vi "Status.vi"(10 "ModuleList":string[](array[string])=["Sync", "FGen", "Digitizer", "Sensor", "Analysis", "Scope", "AcPwr"]) -> ()   [LabVIEW 2018, in "Visualization.lvlib" / "VisualizeStatus.lvclass"]
uses:
  VisualizeStatus.lvclass
  VisualizeBase/VisualizeBase_class/Requests/VisUserEventType.ctl
  <vilib>/event_ctls.llb/usereventprio.ctl
  <extravilib>/ChannelInstances/Tag-bool/Read With Abort.vi
  <extravilib>/ChannelInstances/Tag-bool/Write With Abort.vi
  <vilib>/Utility/error.llb/Error Cluster From Error Code.vi
  <extravilib>/ChannelInstances/Tag-bool/Instantiate.vi
  <extravilib>/ChannelInstances/Tag-bool/EndpointRead.vi
  <extravilib>/ChannelInstances/Tag-bool/Endpoint.vi
  <vilib>/ErrorRing/Error Ring.xnode
  VisualizeBase/VisualizeBase_class/VisualizeBase.lvclass
  <userlib>/NIST/NISTErrorLib/NISTErrorLib.lvlib
  Sync/SyncModule/SyncModule.lvlib
  Digitizer/DigitizerModule/DigitizerModule.lvlib
  BusClass/Bus.lvclass
  Sensor/SensorModule/SensorModule.lvlib
  Analysis/AnalysisModule/AnalysisModule.lvlib
  Scope/ScopeModule/ScopeModule.lvlib
  AcPwr/AcPwrShared/AcPwrShared.lvlib
  <extravilib>/ChannelInstances/Tag-bool.lvlib
  TestClass/Test.lvclass
  FGen/FgenShared/FgenShared.lvlib
panel:
  out "Status Message":string
  out "ErrorArray":errorcluster[](array[cluster])
  in  "btnReset":bool
  in  "btnClear":bool
  in  "QueName":string="StatusVisQue"
  in  "btnStop&Exit":bool
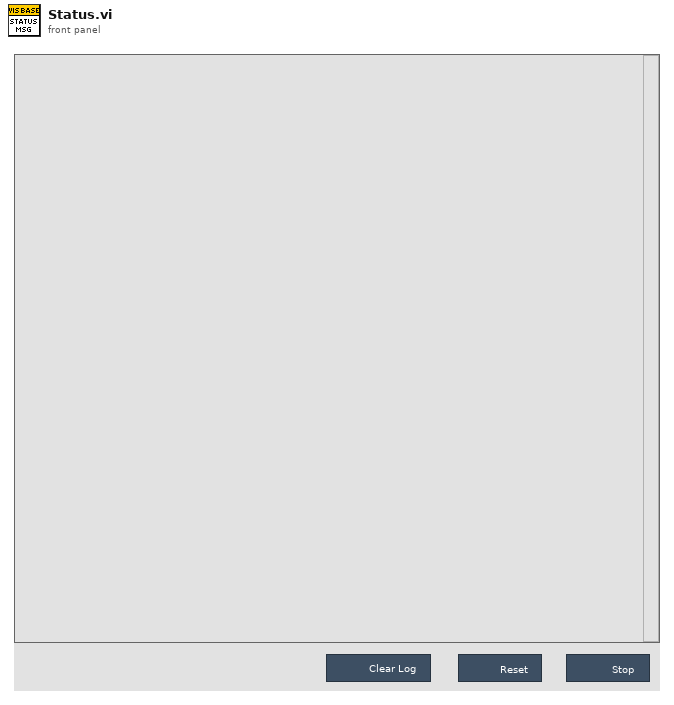
[diagram p1: front panel]
types:
  T1 = typedef "SyncModule.lvlib/SyncBroadcastEvents.ctl" = cluster{"DidInit":refnum<user-event>, "StatusUpdate":refnum<user-event>, "ErrorReport":refnum<user-event>, "DidStop":refnum<user-event>, "PathToINI":refnum<user-event>, "TriggerTime":refnum<user-event>, "LockStatus":refnum<user-event>, "Info":refnum<user-event>, "ClockProperties":refnum<user-event>, "SyncData":refnum<user-event>}
  T2 = typedef "AcPwrShared.lvlib/AcPwrBroadcastEvents.ctl" = cluster{"DidInit":refnum<user-event>, "StatusUpdate":refnum<user-event>, "ErrorReport":refnum<user-event>, "DidStop":refnum<user-event>, "PathToINI":refnum<user-event>, "Measurements":refnum<user-event>, "LoadConfigFile":refnum<user-event>, "GetSettings":refnum<user-event>, "SetSettings":refnum<user-event>, "GetType&ID":refnum<user-event>, "GotSettings":refnum<user-event>}
  T3 = typedef "FgenShared.lvlib/clBroadcastEvents.ctl" = cluster{"DidInit":refnum<user-event>, "StatusUpdate":refnum<user-event>, "ErrorReport":refnum<user-event>, "DidStop":refnum<user-event>, "PathToINI":refnum<user-event>, "Channels":refnum<user-event>, "Function":refnum<user-event>, "Waveforms":refnum<user-event>, "Triggers":refnum<user-event>, "FunctionParams":refnum<user-event>, "FunctionArbs":refnum<user-event>, "FunctionSampleRate":refnum<user-event>}
  T4 = typedef "ScopeShared.lvlib/clBroadcastEvents.ctl" = cluster{"DidInit":refnum<user-event>, "StatusUpdate":refnum<user-event>, "ErrorReport":refnum<user-event>, "DidStop":refnum<user-event>, "PathToINI":refnum<user-event>, "Handle":refnum<user-event>, "Model":refnum<user-event>, "Channels":refnum<user-event>, "Acquisition":refnum<user-event>, "Trigger":refnum<user-event>, "ExtAcquisition":refnum<user-event>, "Waveform":refnum<user-event>}
  T5 = typedef "DigitizerShared.lvlib/clBroadcastEvents.ctl" = cluster{"DidInit":refnum<user-event>, "StatusUpdate":refnum<user-event>, "ErrorReport":refnum<user-event>, "DidStop":refnum<user-event>, "PathToINI":refnum<user-event>, "Channels":refnum<user-event>, "Acq":refnum<user-event>, "Trigger":refnum<user-event>, "Waveforms":refnum<user-event>}
  T6 = typedef "SensorShared.lvlib/clBroadcastEvents.ctl" = cluster{"DidInit":refnum<user-event>, "StatusUpdate":refnum<user-event>, "ErrorReport":refnum<user-event>, "DidStop":refnum<user-event>, "PathToINI":refnum<user-event>, "SensorReport":refnum<user-event>, "SensorConfig":refnum<user-event>}
  T7 = typedef "AnalysisModule.lvlib/clBroadcastEvents.ctl" = cluster{"DidInit":refnum<user-event>, "StatusUpdate":refnum<user-event>, "ErrorReport":refnum<user-event>, "DidStop":refnum<user-event>, "PathToINI":refnum<user-event>, "Config":refnum<user-event>, "ResultReport":refnum<user-event>, "FunctionClass":refnum<user-event>, "State":refnum<user-event>, "FunctionParams":refnum<user-event>, "Duration":refnum<user-event>}
  T8 = cluster{"DigitizerEvents":T5, "FGenEvents":T3, "SyncBroadcastEvents":T1, "AnalysisBroadcastEvents":T7, "SensorBdcstEvents":T6, "ScopeEvents":T4, "clAcPwrEvents":T2}
  T9 = cluster{"StatusUpdate":refnum<user-event>, "ErrorReport":refnum<user-event>, "StatusUpdate":refnum<user-event>, "ErrorReport":refnum<user-event>, "StatusUpdate":refnum<user-event>, "ErrorReport":refnum<user-event>, "StatusUpdate":refnum<user-event>, "ErrorReport":refnum<user-event>, "StatusUpdate":refnum<user-event>, "ErrorReport":refnum<user-event>, "StatusUpdate":refnum<user-event>, "ErrorReport":refnum<user-event>, "FunctionClass":refnum<user-event>, "StatusUpdate":refnum<user-event>, "ErrorReport":refnum<user-event>}
  T10 = typedef "clUserEvents.ctl" = cluster{"StopEvent":refnum<user-event>, "RefreshUserEvents":refnum<user-event>, "StatusUpdate":refnum<user-event>, "RunAllScripts":refnum<user-event>}
  T11 = typedef "Visualization.lvlib/VisualizeBase.lvclass/VisRequestEvents.ctl" = cluster{"StopRequest":refnum<user-event>, "ResetRequest":refnum<user-event>, "FP Pop In or Out":refnum<user-event>}
  T12 = typedef "Visualization.lvlib/VisualizeBase.lvclass/VisUserEventType.ctl" = cluster{"BusIndex":i8, "Data":variant}
  T13 = typedef "usereventprio.ctl" = enum32{"high priority", "normal priority"}
  T14 = typedef "Tag-bool.lvlib/))Channel.ctl" = refnum<queue>
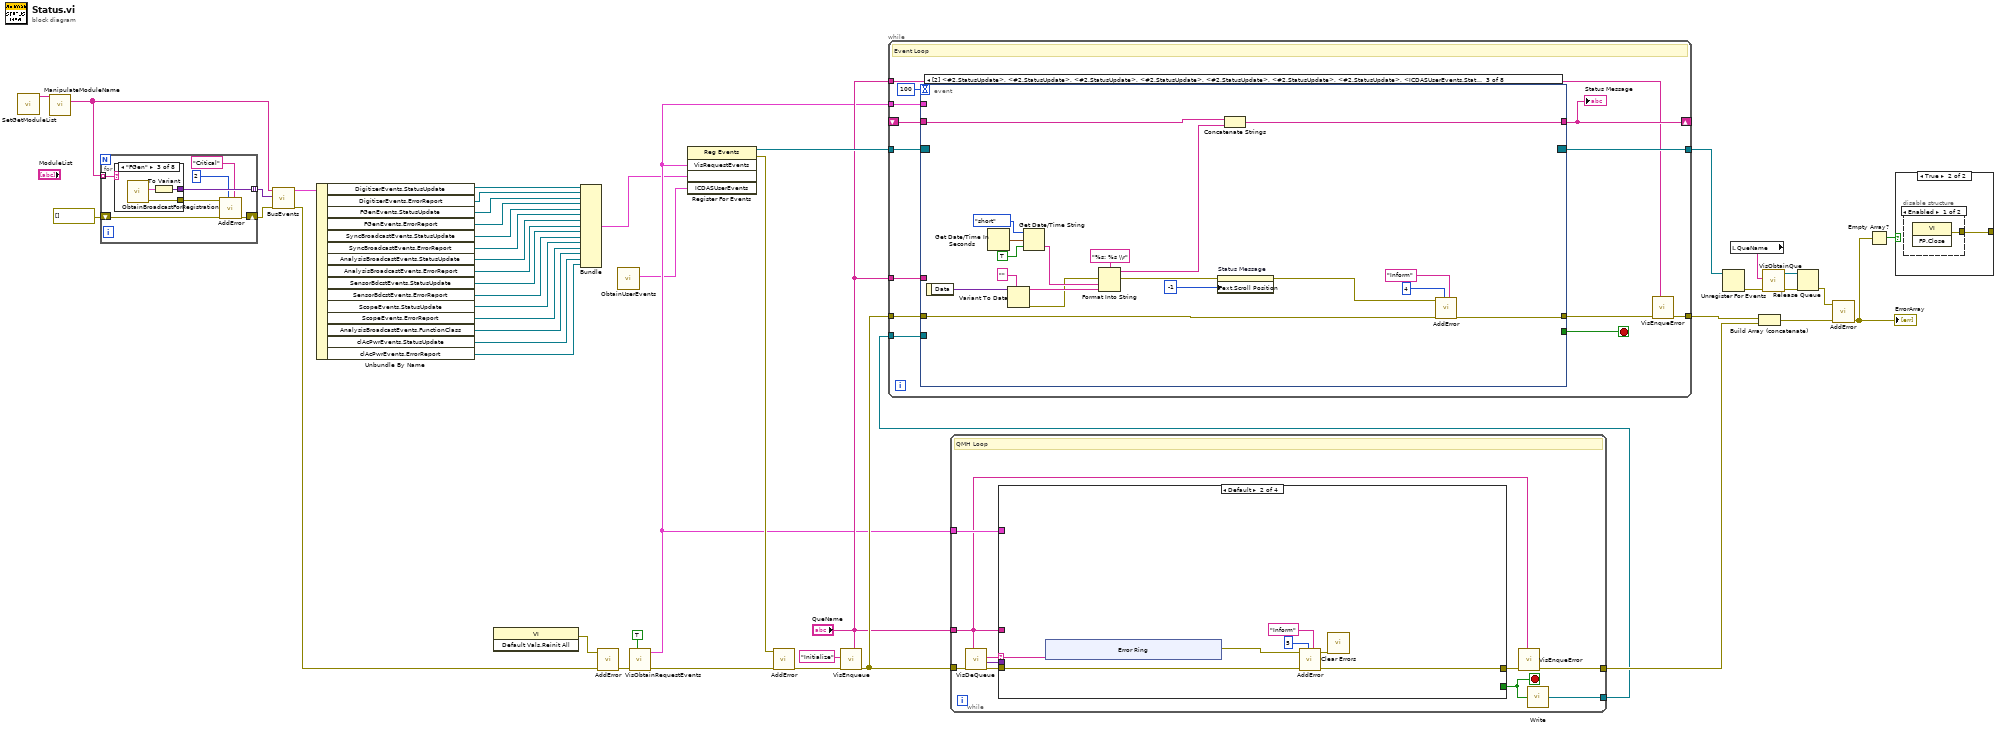
[diagram p0: block diagram]
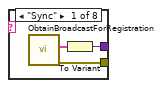
[diagram p2: hidden frame]
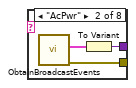
[diagram p3: hidden frame]
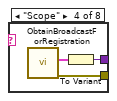
[diagram p4: hidden frame]
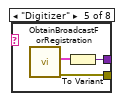
[diagram p5: hidden frame]
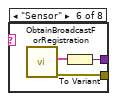
[diagram p6: hidden frame]
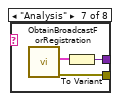
[diagram p7: hidden frame]
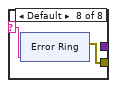
[diagram p8: hidden frame]
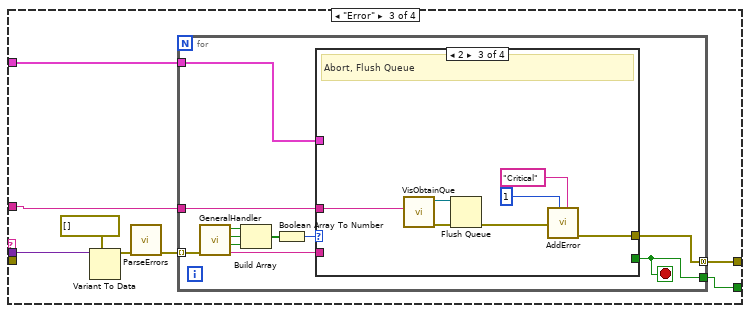
[diagram p10: hidden frame]
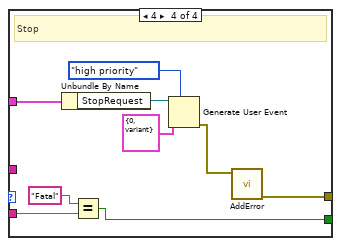
[diagram p13: hidden frame]
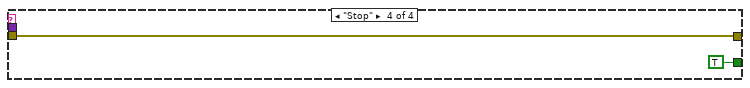
[diagram p14: hidden frame]
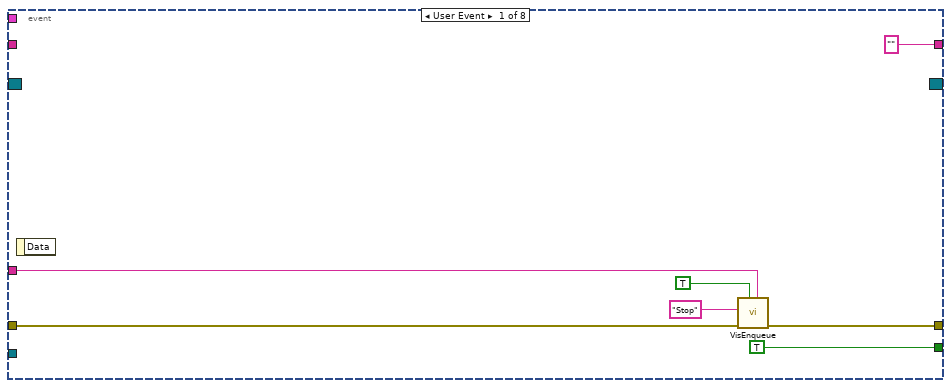
[diagram p15: hidden frame]
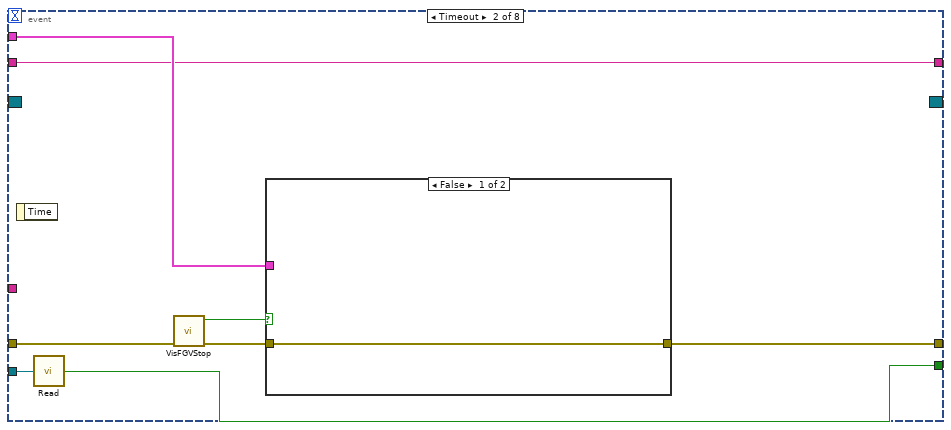
[diagram p16: hidden frame]
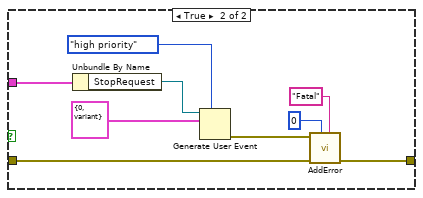
[diagram p17: hidden frame]
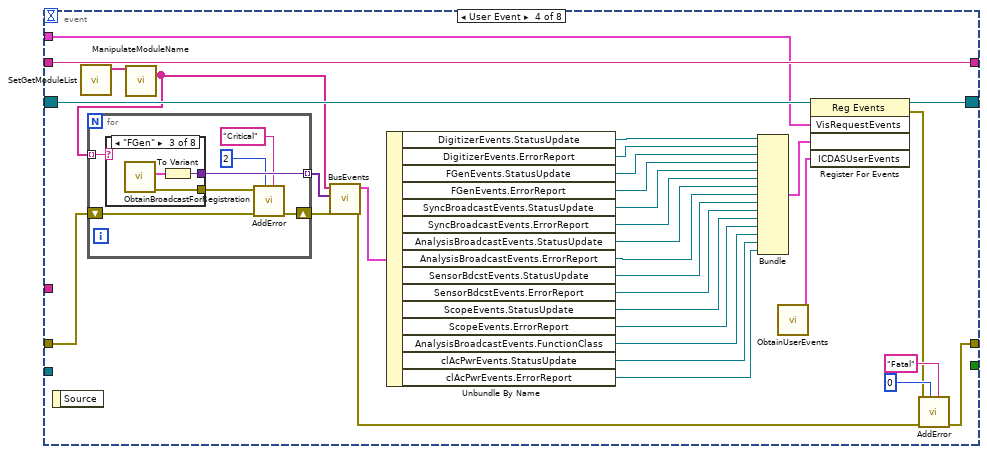
[diagram p18: hidden frame]
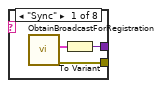
[diagram p19: hidden frame]
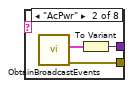
[diagram p20: hidden frame]
diagram:
  n1 = call "SetGetModuleList.vi"() -> ("ModuleList"=w24:string[])  [unwired: 11 in]
  n2 = call "ManipulateModuleName.vi"("ModuleListArrayIn"=w24) -> ("BeforeMatch:ModuleListArray"=w19:string[])  [unwired: 9 in, 5 out]
  n3 = for {
    shift-right: [w52] -> w21
    shift-left: errorcluster[] [] ("ErrorArray") -> [w51]
    tunnel: [w50] -> w20 mode=indexing
    tunnel: w19 -> [w47] mode=indexing
    n4 = case shown="\"FGen\"" w47 {
      selector: w47 -> [_ _ _ _ _ _ _ w75]
      tunnel: [w55 w59 w61 w63 w67 w70 w73 _] -> w50
      tunnel: [w54 w58 w62 w65 w68 w71 w74 w76] -> w53
      frame "Sync" {
        n5 = call "ObtainBroadcastForRegistration.vi"() -> ("error out"=w54:errorcluster, "SyncBroadcastEvents"=w56:T1)  [unwired: 10 in]
        n6 = To Variant(anything=w56) -> (Variant=w55:variant)
      }
      frame "AcPwr" {
        n7 = call "ObtainBroadcastEvents.vi"() -> ("error out"=w58:errorcluster, "clAcPwrEvents"=w57:T2)  [unwired: 10 in]
        n8 = To Variant(anything=w57) -> (Variant=w59:variant)
      }
      frame "FGen" {
        n9 = call "ObtainBroadcastForRegistration.vi"() -> ("error out"=w62:errorcluster, "FgenBroadcastEvents"=w60:T3)  [unwired: 10 in]
        n10 = To Variant(anything=w60) -> (Variant=w61:variant)
      }
      frame "Scope" {
        n11 = call "ObtainBroadcastForRegistration.vi"() -> ("error out"=w65:errorcluster, "ScopeBroadcastEvents"=w64:T4)  [unwired: 10 in]
        n12 = To Variant(anything=w64) -> (Variant=w63:variant)
      }
      frame "Digitizer" {
        n13 = call "ObtainBroadcastForRegistration.vi"() -> ("error out"=w68:errorcluster, "clDigitizerBdcstEvents"=w66:T5)  [unwired: 10 in]
        n14 = To Variant(anything=w66) -> (Variant=w67:variant)
      }
      frame "Sensor" {
        n15 = call "ObtainBroadcastForRegistration.vi"() -> ("error out"=w71:errorcluster, "SensorBdcstEvents"=w69:T6)  [unwired: 10 in]
        n16 = To Variant(anything=w69) -> (Variant=w70:variant)
      }
      frame "Analysis" {
        n17 = call "ObtainBroadcastForRegistration.vi"() -> ("error out"=w74:errorcluster, "AnalysisBroadcastEvents"=w72:T7)  [unwired: 10 in]
        n18 = To Variant(anything=w72) -> (Variant=w73:variant)
      }
      frame Default {
        n19 = xnode "Error Ring"("parameter 0"=w75) -> ("error out"=w76:errorcluster)
      }
    }
    n20 = call <userlib>:"AddError.vi"("Severity"="Critical", "Priority"=u8 2, "ErrorArray In"=w51, "error in (no error)"=w53) -> ("ErrorArray Out"=w52:errorcluster[])  [unwired: 6 in, 1 out]
  }
  n21 = call "BusEvents.vi"("Error in"=w21, "EventArray"=w20, "ModuleList"=w19) -> ("output cluster"=w18:T8)  [unwired: 7 in, 1 out]
  n22 = Unbundle By Name(w18) -> ("DigitizerEvents.StatusUpdate"=w17:refnum<user-event>, "DigitizerEvents.ErrorReport"=w16:refnum<user-event>, "FGenEvents.StatusUpdate"=w15:refnum<user-event>, "FGenEvents.ErrorReport"=w14:refnum<user-event>, "SyncBroadcastEvents.StatusUpdate"=w13:refnum<user-event>, "SyncBroadcastEvents.ErrorReport"=w12:refnum<user-event>, "AnalysisBroadcastEvents.StatusUpdate"=w11:refnum<user-event>, "AnalysisBroadcastEvents.ErrorReport"=w10:refnum<user-event>, "SensorBdcstEvents.StatusUpdate"=w9:refnum<user-event>, "SensorBdcstEvents.ErrorReport"=w8:refnum<user-event>, "ScopeEvents.StatusUpdate"=w7:refnum<user-event>, "ScopeEvents.ErrorReport"=w6:refnum<user-event>, "AnalysisBroadcastEvents.FunctionClass"=w5:refnum<user-event>, "clAcPwrEvents.StatusUpdate"=w4:refnum<user-event>, "clAcPwrEvents.ErrorReport"=w3:refnum<user-event>)
  n23 = invoke class="VI" method="Default Vals.Reinit All"() -> (error out=w45:errorcluster)  [unwired: 3 in, 2 out]
  n24 = Bundle("StatusUpdate"=w17, "ErrorReport"=w16, "StatusUpdate"=w15, "ErrorReport"=w14, "StatusUpdate"=w13, "ErrorReport"=w12, "StatusUpdate"=w11, "ErrorReport"=w10, "StatusUpdate"=w9, "ErrorReport"=w8, "StatusUpdate"=w7, "ErrorReport"=w6, "FunctionClass"=w5, "StatusUpdate"=w4, "ErrorReport"=w3) -> (w2:T9)  [unwired: 1 in]
  n25 = call <userlib>:"AddError.vi"("ErrorArray In"=w21, "error in (no error)"=w45) -> ("ErrorArray Out"=w44:errorcluster[])  [unwired: 8 in, 1 out]
  n26 = call "ObtainUserEvents.vi"() -> ("ICDASUserEvents"=w22:T10)  [unwired: 10 in, 1 out]
  n27 = call "VisObtainRequestEvents.vi"("Set (T)/Get (F)"=TRUE, "Error"=w44) -> ("Error"=w43:errorcluster[], "VisRequestEvents"=w25:T11)  [unwired: 8 in]
  n28 = register-events(w25, w2, w22) -> (reference out=w31:refnum<event-registration>, error out=w30:errorcluster)  [unwired: 2 in]
  n29 = call <userlib>:"AddError.vi"("ErrorArray In"=w43, "error in (no error)"=w30) -> ("ErrorArray Out"=w32:errorcluster[])  [unwired: 8 in, 1 out]
  n30 = call "VisEnqueue.vi"("QueName"="QueName", "Error"=w32, "Message"="Initialize") -> ("Error"=w28:errorcluster[])  [unwired: 8 in]
  n31 = while {
    tunnel: w28 -> [w93]
    tunnel: [w87] -> w40
    tunnel: w25 -> [w86]
    tunnel: "QueName" -> [w85]
    tunnel: [w84] -> w26
    stop <- w88 stop-if-true
    # "QMH Loop"
    n32 = call "VisDeQueue.vi"("QueName"=w85, "Error"=w93) -> ("Error"=w90:errorcluster[], "Data"=w91:variant, "Message"=w92:string)  [unwired: 7 in]
    n33 = case shown="Default" w92 {
      selector: w92 -> [_ w101 _ _]
      tunnel: w91 -> [_ _ w116 _]
      tunnel: w90 -> [w94 w99 _ w144]
      tunnel: [w94 w98 w112 w144] -> w89
      tunnel: [_ _ w111 TRUE] -> w88
      tunnel: w86 -> [_ _ w110 _]
      tunnel: w85 -> [_ _ w109 _]
      frame "Initialize" {
      }
      frame Default {
        n34 = xnode "Error Ring"("parameter 0"=w101) -> ("error out"=w100:errorcluster)
        n35 = call <userlib>:"AddError.vi"("Severity"="Inform" ("String"), "Priority"=u8 5, "ErrorArray In"=w99, "error in (no error)"=w100) -> ("ErrorArray Out"=w98:errorcluster[], "error out"=w97:errorcluster)  [unwired: 6 in]
        n36 = call <vilib>:"Clear Errors.vi"("error in (no error)"=w97) -> ()  [unwired: 5 in, 2 out]
      }
      frame "Error" {
        n37 = Variant To Data(type=errorcluster[] [], Variant=w116) -> (data=w114:errorcluster[])  [unwired: 1 in, 1 out]
        n38 = call <userlib>:"ParseErrors.vi"("ErrorArray"=w114) -> ("ErrorArray"=w113:errorcluster[])  [unwired: 8 in, 2 out]
        n39 = for {
          tunnel: w113 -> [w127] mode=indexing
          tunnel: [w121] -> w112 mode=concatenating
          tunnel: [w119] -> w111
          tunnel: w110 -> [w118]
          tunnel: w109 -> [w117]
          stop <- w119 stop-if-true
          n40 = call <userlib>:"GeneralHandler.vi"("error in (no error)"=w127) -> ("Severity"=w120:string, "Stop"=w124:bool, "Abort"=w125:bool, "Continue"=w126:bool)  [unwired: 6 in, 1 out]
          n41 = Build Array(w126, w125, w124) -> (w123:bool[])
          n42 = Boolean Array To Number(Boolean array=w123) -> (number=w122:u32)
          n43 = case shown="2" w122 {
            tunnel: [_ _ w132 w142] -> w121
            tunnel: w120 -> [_ _ _ w138]
            tunnel: [_ _ _ w136] -> w119
            tunnel: w118 -> [_ _ _ w135]
            tunnel: w117 -> [_ _ w128 _]
            frame 0, Default {
              # "No Dialog"
            }
            frame 1 {
              # "Continue"
            }
            frame 2 {
              # "Abort, Flush Queue"
              n44 = call "VisObtainQue.vi"("QueName"=w128) -> ("error out"=w134:errorcluster, "queue out"=w133:refnum<queue>)  [unwired: 9 in]
              n45 = Flush Queue(queue=w133, error in (no error)=w134) -> (error out=w131:errorcluster)  [unwired: 2 out]
              n46 = call <userlib>:"AddError.vi"("Severity"="Critical" ("String"), "Priority"=u8 1, "error in (no error)"=w131) -> ("ErrorArray Out"=w132:errorcluster[])  [unwired: 7 in, 1 out]
            }
            frame 4 {
              # "Stop"
              n47 = Unbundle By Name(w135) -> ("StopRequest"=w143:refnum<user-event>)
              n48 = Equal?(x="Fatal", y=w138) -> (x = y?=w136:bool)
              n49 = Generate User Event(priority (normal)=usereventprio."high priority", user event=w143, event data cluster=T12 {"BusIndex"=0, "Data"=variant} ("event data")) -> (error out=w141:errorcluster)  [unwired: 1 in, 1 out]
              n50 = call <userlib>:"AddError.vi"("error in (no error)"=w141) -> ("ErrorArray Out"=w142:errorcluster[])  [unwired: 9 in, 1 out]
            }
          }
        }
      }
      frame "Stop" {
      }
    }
    n51 = call "VisEnqueError.vi"("QueName"=w85, "Error"=w89) -> ("Error"=w87:errorcluster[])  [unwired: 9 in]
    n52 = call <extravilib>:"Write.vi"("element"=w88) -> ("channel"=w84:T14)  [unwired: 1 out]
  }
  n53 = while {
    tunnel: w31 -> [w158]
    tunnel: [w155] -> w41
    tunnel: [w154] -> w42
    tunnel: w25 -> [w153]
    shift-right: [w150] -> _
    shift-left: _ -> [w152]
    tunnel: w28 -> [w151]
    tunnel: "QueName" -> [w149]
    tunnel: "QueName" -> [w148]
    tunnel: w26 -> [w146]
    stop <- w157 stop-if-true
    # "Event Loop"
    n54 = event shown="[2] <#2.StatusUpdate>, <#2.StatusUpdate>, <#2.StatusUpdate>, <#2.StatusUpdate>, <#2.StatusUpdate>, <#2.StatusUpdate>, <#2.StatusUpdate>, <ICDASUserEvents.StatusUpdate>: User Event" {
      selector: w158 -> [_ _ _ w229 _ _ _ _]
      dyn-events: [_ _ _ w231 _ _ _ _] -> w154
      timeout: 100 -> [_ _ _ _ _ _ _ _]
      tunnel: [TRUE w166 _ _ _ _ _ _] -> w157
      tunnel: [w164 w172 w194 w234 w281 _ w300 w306] -> w156
      tunnel: w153 -> [_ w169 _ w222 _ _ w295 w305]
      tunnel: ["" w168 w190 w227 w276 "" w293 w303] -> w150
      tunnel: w152 -> [_ w168 w189 w227 w275 _ w293 w303]
      tunnel: w151 -> [w160 w171 w188 w228 w272 _ w294 w304]
      tunnel: w148 -> [w161 _ _ _ _ _ _ _]
      tunnel: w146 -> [_ w167 _ _ _ _ _ _]
      event User Event {
        n55 = event-data() -> ()  [unwired: 1 in, 1 out]
        n56 = call "VisEnqueue.vi"("QueName"=w161, "Priority? (F)"=TRUE, "Error"=w160, "Message"="Stop") -> ("Error"=w164:errorcluster[])  [unwired: 7 in]
      }
      event Timeout {
        n57 = event-data() -> ()  [unwired: 1 in, 1 out]
        n58 = call <extravilib>:"Read.vi"("channel"=w167) -> ("element"=w166:bool)  [unwired: 1 in, 1 out]
        n59 = call "VisFGVStop.vi"("Error In"=w171) -> ("Error Out"=w170:errorcluster[], "Value"=w173:bool)  [unwired: 9 in]
        n60 = case shown="False" w173 {
          tunnel: [w174 w177] -> w172
          tunnel: w170 -> [w174 w176]
          tunnel: w169 -> [_ w175]
          frame False {
          }
          frame True {
            n61 = Unbundle By Name(w175) -> ("StopRequest"=w183:refnum<user-event>)
            n62 = Generate User Event(priority (normal)=usereventprio."high priority", user event=w183, event data cluster=T12 {"BusIndex"=0, "Data"=variant} ("event data")) -> (error out=w178:errorcluster)  [unwired: 1 in, 1 out]
            n63 = call <userlib>:"AddError.vi"("Severity"="Fatal" ("String"), "Priority"=u8 0, "ErrorArray In"=w176, "error in (no error)"=w178) -> ("ErrorArray Out"=w177:errorcluster[])  [unwired: 6 in, 1 out]
          }
        }
      }
      event User Event {
        n64 = event-data() -> ("Data"=w184:variant)  [unwired: 1 in]
        n65 = Get Date/Time In Seconds() -> (seconds since 1Jan1904=w202:timestamp)
        n66 = Variant To Data(type="", Variant=w184) -> (data=w196:string, error out=w195:errorcluster)  [unwired: 1 in]
        n67 = Get Date/Time String(date format (0)=enum16{"short", "long", "abbreviated"}."short", seconds (now)=w202, want seconds? (F)=TRUE) -> (time string=w197:string)  [unwired: 1 out]
        n68 = Format Into String(format string="%s: %s \\r", error in=w195, w197, w196) -> (resulting string=w191:string, error out=w187:errorcluster)  [unwired: 1 in]
        n69 = property on="Status Message" class="Str"(error in=w187, "Text.Scroll Position"=-1) -> (error out=w186:errorcluster)  [unwired: 1 in, 1 out]
        n70 = Concatenate Strings(w189, w191) -> (w190:string)
        n71 = call <userlib>:"AddError.vi"("Severity"="Inform", "Priority"=u8 4, "ErrorArray In"=w188, "error in (no error)"=w186) -> ("ErrorArray Out"=w194:errorcluster[])  [unwired: 6 in, 1 out]
      }
      event User Event {
        n72 = event-data() -> ()  [unwired: 1 in, 1 out]
        n73 = call "SetGetModuleList.vi"() -> ("ModuleList"=w226:string[])  [unwired: 11 in]
        n74 = call "ManipulateModuleName.vi"("ModuleListArrayIn"=w226) -> ("BeforeMatch:ModuleListArray"=w203:string[])  [unwired: 9 in, 5 out]
        n75 = for {
          shift-right: [w240] -> w223
          shift-left: w228 -> [w239]
          tunnel: [w238] -> w225 mode=indexing
          tunnel: w203 -> [w235] mode=indexing
          n76 = case shown="\"FGen\"" w235 {
            selector: w235 -> [_ _ _ _ _ _ _ w263]
            tunnel: [w243 w247 w249 w253 w255 w258 w261 _] -> w238
            tunnel: [w242 w246 w250 w252 w256 w259 w262 w264] -> w241
            frame "Sync" {
              n77 = call "ObtainBroadcastForRegistration.vi"() -> ("error out"=w242:errorcluster, "SyncBroadcastEvents"=w244:T1)  [unwired: 10 in]
              n78 = To Variant(anything=w244) -> (Variant=w243:variant)
            }
            frame "AcPwr" {
              n79 = call "ObtainBroadcastEvents.vi"() -> ("error out"=w246:errorcluster, "clAcPwrEvents"=w245:T2)  [unwired: 10 in]
              n80 = To Variant(anything=w245) -> (Variant=w247:variant)
            }
            frame "FGen" {
              n81 = call "ObtainBroadcastForRegistration.vi"() -> ("error out"=w250:errorcluster, "FgenBroadcastEvents"=w248:T3)  [unwired: 10 in]
              n82 = To Variant(anything=w248) -> (Variant=w249:variant)
            }
            frame "Scope" {
              n83 = call "ObtainBroadcastForRegistration.vi"() -> ("error out"=w252:errorcluster, "ScopeBroadcastEvents"=w251:T4)  [unwired: 10 in]
              n84 = To Variant(anything=w251) -> (Variant=w253:variant)
            }
            frame "Digitizer" {
              n85 = call "ObtainBroadcastForRegistration.vi"() -> ("error out"=w256:errorcluster, "clDigitizerBdcstEvents"=w254:T5)  [unwired: 10 in]
              n86 = To Variant(anything=w254) -> (Variant=w255:variant)
            }
            frame "Sensor" {
              n87 = call "ObtainBroadcastForRegistration.vi"() -> ("error out"=w259:errorcluster, "SensorBdcstEvents"=w257:T6)  [unwired: 10 in]
              n88 = To Variant(anything=w257) -> (Variant=w258:variant)
            }
            frame "Analysis" {
              n89 = call "ObtainBroadcastForRegistration.vi"() -> ("error out"=w262:errorcluster, "AnalysisBroadcastEvents"=w260:T7)  [unwired: 10 in]
              n90 = To Variant(anything=w260) -> (Variant=w261:variant)
            }
            frame Default {
              n91 = xnode "Error Ring"("parameter 0"=w263) -> ("error out"=w264:errorcluster)
            }
          }
          n92 = call <userlib>:"AddError.vi"("Severity"="Critical", "Priority"=u8 2, "ErrorArray In"=w239, "error in (no error)"=w241) -> ("ErrorArray Out"=w240:errorcluster[])  [unwired: 6 in, 1 out]
        }
        n93 = call "BusEvents.vi"("Error in"=w223, "EventArray"=w225, "ModuleList"=w203) -> ("Error out"=w224:errorcluster[], "output cluster"=w220:T8)  [unwired: 7 in]
        n94 = Unbundle By Name(w220) -> ("DigitizerEvents.StatusUpdate"=w219:refnum<user-event>, "DigitizerEvents.ErrorReport"=w218:refnum<user-event>, "FGenEvents.StatusUpdate"=w217:refnum<user-event>, "FGenEvents.ErrorReport"=w216:refnum<user-event>, "SyncBroadcastEvents.StatusUpdate"=w215:refnum<user-event>, "SyncBroadcastEvents.ErrorReport"=w214:refnum<user-event>, "AnalysisBroadcastEvents.StatusUpdate"=w213:refnum<user-event>, "AnalysisBroadcastEvents.ErrorReport"=w212:refnum<user-event>, "SensorBdcstEvents.StatusUpdate"=w211:refnum<user-event>, "SensorBdcstEvents.ErrorReport"=w210:refnum<user-event>, "ScopeEvents.StatusUpdate"=w209:refnum<user-event>, "ScopeEvents.ErrorReport"=w208:refnum<user-event>, "AnalysisBroadcastEvents.FunctionClass"=w207:refnum<user-event>, "clAcPwrEvents.StatusUpdate"=w206:refnum<user-event>, "clAcPwrEvents.ErrorReport"=w205:refnum<user-event>)
        n95 = Bundle("StatusUpdate"=w219, "ErrorReport"=w218, "StatusUpdate"=w217, "ErrorReport"=w216, "StatusUpdate"=w215, "ErrorReport"=w214, "StatusUpdate"=w213, "ErrorReport"=w212, "StatusUpdate"=w211, "ErrorReport"=w210, "StatusUpdate"=w209, "ErrorReport"=w208, "FunctionClass"=w207, "StatusUpdate"=w206, "ErrorReport"=w205) -> (w204:T9)  [unwired: 1 in]
        n96 = call "ObtainUserEvents.vi"() -> ("ICDASUserEvents"=w221:T10)  [unwired: 10 in, 1 out]
        n97 = register-events(reference=w229, w222, w204, w221) -> (reference out=w231:refnum<event-registration>, error out=w230:errorcluster)  [unwired: 1 in]
        n98 = call <userlib>:"AddError.vi"("Severity"="Fatal", "Priority"=u8 0, "ErrorArray In"=w224, "error in (no error)"=w230) -> ("ErrorArray Out"=w234:errorcluster[])  [unwired: 6 in, 1 out]
      }
      event User Event {
        n99 = event-data() -> ("Data"=w288:variant)  [unwired: 1 in]
        n100 = Get Date/Time In Seconds() -> (seconds since 1Jan1904=w291:timestamp)
        n101 = Variant To Data(type=errorcluster {"status"=FALSE, "code"=0, "source"=""} ("error constant"), Variant=w288) -> (data=w285:errorcluster, error out=w284:errorcluster)  [unwired: 1 in]
        n102 = Get Date/Time String(date format (0)=enum16{"short", "long", "abbreviated"}."short", seconds (now)=w291, want seconds? (F)=TRUE) -> (time string=w286:string)  [unwired: 1 out]
        n103 = Unbundle By Name(w285) -> ("source"=w273:string)
        n104 = Format Into String(format string="%s: %s \\r", error in=w284, w286, w273) -> (resulting string=w277:string, error out=w283:errorcluster)  [unwired: 1 in]
        n105 = property on="Status Message" class="Str"(error in=w283, "Text.Scroll Position"=-1) -> (error out=w280:errorcluster)  [unwired: 1 in, 1 out]
        n106 = Concatenate Strings(w275, w277) -> (w276:string)
        n107 = call <userlib>:"AddError.vi"("Severity"="Inform", "Priority"=u8 4, "ErrorArray In"=w272, "error in (no error)"=w280) -> ("ErrorArray Out"=w281:errorcluster[])  [unwired: 6 in, 1 out]
      }
      event "btnClear": Value Change {
        n108 = event-data() -> ()  [unwired: 1 in, 1 out]
      }
      event "btnStop&Exit": Value Change; User Event {
        n109 = event-data() -> ()  [unwired: 1 in, 1 out]
        n110 = Unbundle By Name(w295) -> ("StopRequest"=w301:refnum<user-event>)
        n111 = Generate User Event(priority (normal)=usereventprio."high priority", user event=w301, event data cluster=T12 {"BusIndex"=0, "Data"=variant} ("event data")) -> (error out=w302:errorcluster)  [unwired: 1 in, 1 out]
        n112 = call <userlib>:"AddError.vi"("Severity"="Inform" ("String"), "Priority"=u8 0, "ErrorArray In"=w294, "error in (no error)"=w302) -> ("ErrorArray Out"=w300:errorcluster[])  [unwired: 6 in, 1 out]
      }
      event "btnReset": Value Change {
        n113 = event-data() -> ()  [unwired: 1 in, 1 out]
        n114 = Unbundle By Name(w305) -> ("ResetRequest"=w307:refnum<user-event>)
        n115 = Generate User Event(priority (normal)=usereventprio."high priority", user event=w307, event data cluster=T12 {"BusIndex"=0, "Data"=variant} ("event data")) -> (error out=w310:errorcluster)  [unwired: 1 in, 1 out]
        n116 = call <userlib>:"AddError.vi"("Severity"="Fatal", "Priority"=u8 0, "ErrorArray In"=w304, "error in (no error)"=w310) -> ("ErrorArray Out"=w306:errorcluster[])  [unwired: 6 in, 1 out]
      }
    }
    "Status Message" <- w150
    n117 = call "VisEnqueError.vi"("QueName"=w149, "Error"=w156) -> ("Error"=w155:errorcluster[])  [unwired: 9 in]
  }
  n118 = Unregister For Events(event registration refnum=w42) -> (error out=w39:errorcluster)  [unwired: 1 in]
  n119 = local read "QueName"() -> (w38:string)
  n120 = Build Array (concatenate)(w41, w40) -> (w37:errorcluster[])
  n121 = call "VisObtainQue.vi"("error in (no error)"=w39, "QueName"=w38) -> ("error out"=w36:errorcluster, "queue out"=w35:refnum<queue>)  [unwired: 8 in]
  n122 = Release Queue(queue=w35, error in (no error)=w36) -> (error out=w34:errorcluster)  [unwired: 1 in, 2 out]
  n123 = call <userlib>:"AddError.vi"("ErrorArray In"=w37, "error in (no error)"=w34) -> ("ErrorArray Out"=w1:errorcluster[])  [unwired: 8 in, 1 out]
  "ErrorArray" <- w1
  n124 = Empty Array?(array=w1) -> (empty?=w33:bool)
  n125 = case shown="True" w33 {
    tunnel: [_ w313] -> _
    frame False {
    }
    frame True {
      n126 = disable-structure shown="Enabled" {
        disable-tunnel: [w314 _] -> w313
        frame Enabled {
          n127 = invoke class="VI" method="FP.Close"() -> (error out=w314:errorcluster)  [unwired: 3 in, 2 out]
        }
        frame Disabled {
        }
      }
    }
  }
